vi "RP Lock-in Test.vi"() -> ()   [LabVIEW 2016]
uses:
  Instruments/Instrument Driver/Lock-in Driver/Lock-in Configuration.ctl
  Red Pitaya Lock-in Driver.lvclass
  C:/github/NHMFL_Core/Libraries/Instruments/Instrument Driver/Lock-in Driver/Lock-in Driver.lvclass
  C:/github/NHMFL_Core/Libraries/Instruments/Instrument Driver/Instrument Driver.lvclass
  Instruments/Instrument Driver/Instrument Driver.lvclass/Instrument Driver.ctl
  Red Pitaya Lock-in Driver.lvclass/Red Pitaya Lock-in Driver.ctl
  Instruments/Instrument Driver/Read Cycle period.vi
  Instruments/Instrument Driver/Read Group name.vi
  Instruments/Instrument Driver/Read Channel names.vi
  Instruments/Instrument Driver/Write Recorder name.vi
  Instruments/Instrument Driver/Write Cycle period.vi
  Read RP Instrument.vi
  Write RP Instrument.vi
  Instruments/Instrument Driver/Lock-in Driver/Write Lock-in configuration.vi
  RP Instrument/Write Server address.vi
  RP Instrument/Write Client type.vi
  Instruments/Instrument Driver/Lock-in Driver/Read Lock-in configuration.vi
  RP Instrument/RP Instrument.lvclass
  Instruments/Results/Acquired Result/Acquired Result.lvclass
panel:
  in  "Save result":bool
  in  "File Path Control":path=path "C:/Data/RPtest.tdms"
  out "XY Graph":cluster{dbl[], dbl[]}[](graph)
  in  "Update period":dbl=0.001 format="%#_6ps"
  in  "Lock-in configuration":T1={"Frequency"=0.0, "Time constant"=0.001, "Synchronous"=FALSE, "Channels"=[1]} {"Time constant" format="%#_6ps"; "Frequency" format="%#_6pHz"}
  in  "Start":dbl=1000.0 format="%#_6pHz"
  in  "End":dbl=10000000.0 format="%#_6pHz"
  in  "Step":dbl=10000.0 format="%#_6pHz"
  in  "Server address":string="192.168.1.100"
  out "Error Out":errorcluster
  in  "Error In":errorcluster
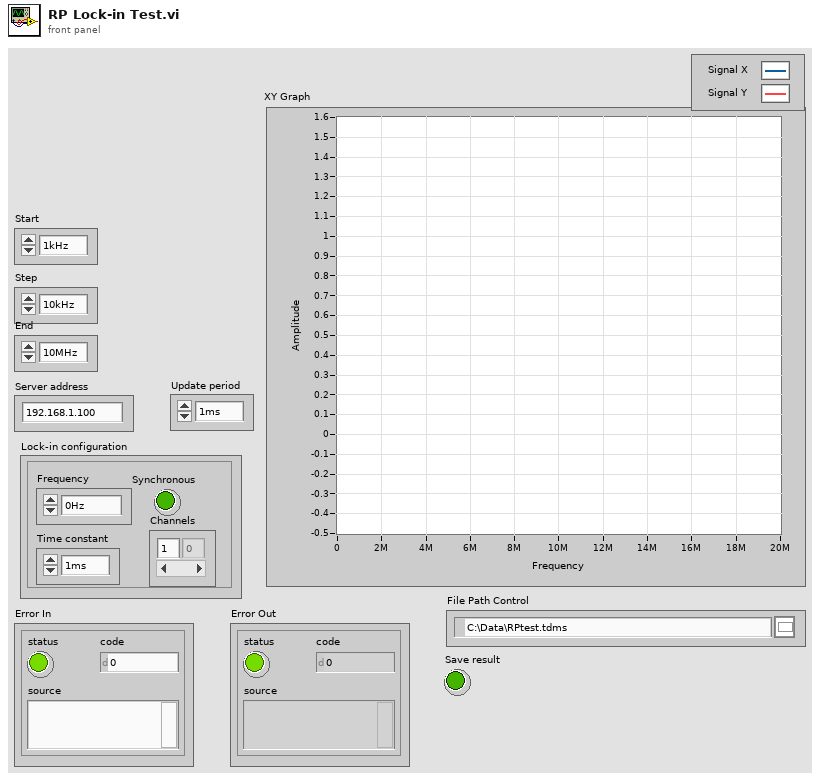
[diagram p1: front panel]
types:
  T1 = typedef "Lock-in Configuration.ctl" = cluster{"Frequency":dbl, "Time constant":dbl, "Synchronous":bool, "Channels":i32[]}
  T2 = enum16{"open", "open or create", "create or replace", "create", "open (read-only)"}
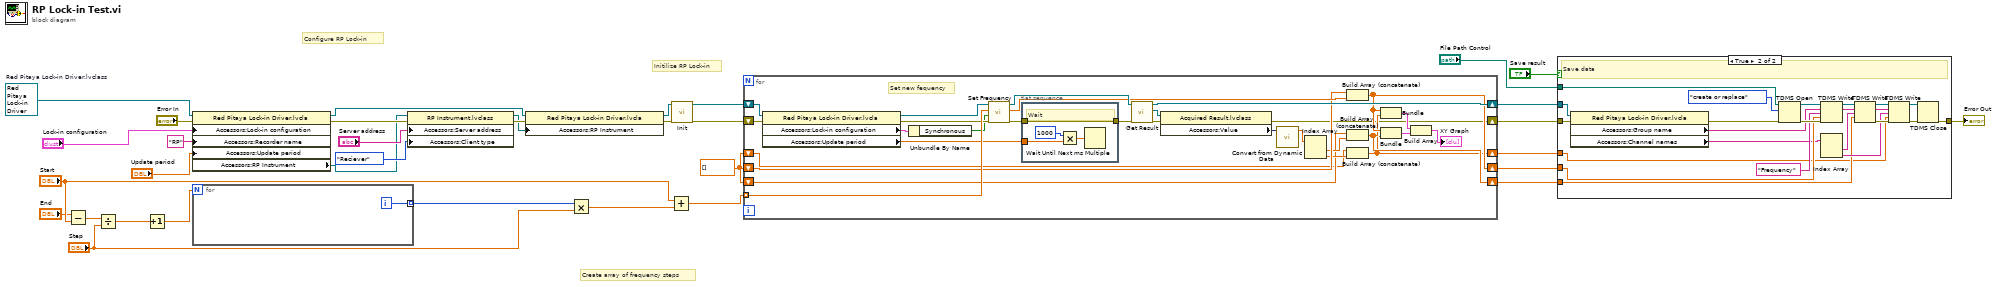
[diagram p0: block diagram]
diagram:
  w9 = dbl[] []
  w33 = refnum<class "Red Pitaya Lock-in Driver.lvclass"> refnum  # Red Pitaya Lock-in Driver.lvclass
  # "Initilize RP Lock-in"
  # "Configure RP Lock-in"
  # "Create array of frequency steps"
  n1 = Subtract(x="End", y="Start") -> (x-y=w20:dbl)
  n2 = Divide(x=w20, y="Step") -> (x/y=w21:dbl)
  n3 = Increment(x=w21) -> (x+1=w22:dbl)
  n4 = property class="Red Pitaya Lock-in Driver.lvcla"(reference=w33, error in="Error In", "Accessors:Lock-in configuration"="Lock-in configuration", "Accessors:Recorder name"="RP" ("Recorder name"), "Accessors:Update period"="Update period") -> (reference out=w29:refnum<class "Red Pitaya Lock-in Driver.lvclass">, error out=w31:errorcluster, "Accessors:RP Instrument"=w13:refnum<class "RP Instrument.lvclass">)
  n5 = for {
    N: w22 -> [_]
    tunnel: [w35] -> w23 mode=indexing
    i -> [w35]
  }
  n6 = property class="RP Instrument.lvclass"(reference=w13, error in=w31, "Accessors:Server address"="Server address", "Accessors:Client type"=enum16{"Control", "Reciever", "Transmitter"}."Reciever" ("Client type")) -> (reference out=w30:refnum<class "RP Instrument.lvclass">, error out=w32:errorcluster)
  n7 = property class="Red Pitaya Lock-in Driver.lvcla"(reference=w29, error in=w32, "Accessors:RP Instrument"=w30) -> (reference out=w16:refnum<class "Red Pitaya Lock-in Driver.lvclass">, error out=w17:errorcluster)
  n8 = Multiply(x=w23, y="Step") -> (x*y=w25:dbl[])
  n9 = Add(x="Start", y=w25) -> (x+y=w18:dbl[])
  n10 = call-dynamic "Init.vi"("error in (no error)"=w17, "Instrument Driver in"=w16) -> ("error out"=w14:errorcluster, "Instrument Driver out"=w15:refnum<class "Red Pitaya Lock-in Driver.lvclass">)  [unwired: 7 in, 1 out]
  n11 = for {
    tunnel: w18 -> [w64] mode=indexing
    shift-right: [w36] -> w7
    shift-left: w14 -> [w63]
    shift-right: [w52] -> w5
    shift-left: w15 -> [w61]
    shift-right: [w45] -> w4
    shift-left: w9 -> [w46]
    shift-right: [w38] -> w3
    shift-left: w9 -> [w40]
    shift-right: [w37] -> w2
    shift-left: w9 -> [w39]
    # "Set new fequency"
    n12 = property class="Red Pitaya Lock-in Driver.lvcla"(reference=w61, error in=w63) -> (reference out=w60:refnum<class "Red Pitaya Lock-in Driver.lvclass">, error out=w62:errorcluster, "Accessors:Lock-in configuration"=w59:T1, "Accessors:Update period"=w57:dbl)
    n13 = Unbundle By Name(w59) -> ("Synchronous"=w58:bool)
    n14 = call-dynamic "Set Frequency.vi"("error in (no error)"=w62, "Synchronous"=w58, "Frequency"=w64, "Red Pitaya Lock-in Driver in"=w60) -> ("error out"=w56:errorcluster, "Actual frequency"=w47:dbl, "Red Pitaya Lock-in Driver out"=w54:refnum<class "Red Pitaya Lock-in Driver.lvclass">)  [unwired: 5 in]
    n15 = flat-sequence {
      tunnel: w57 -> [w68]
      tunnel: w56 -> [w65]
      tunnel: [w65] -> w55
      frame #0 {
        # "Wait"
        n16 = Multiply(x=1000, y=w68) -> (x*y=w67:dbl)
        n17 = Wait Until Next ms Multiple(millisecond multiple=w67) -> ()  [unwired: 1 out]
      }
    }
    n18 = call-dynamic "Get Result.vi"("error in (no error)"=w55, "Red Pitaya Lock-in Driver in"=w54) -> ("error out"=w51:errorcluster, "Result"=w53:refnum<class "Acquired Result.lvclass">, "Red Pitaya Lock-in Driver out"=w52:refnum<class "Red Pitaya Lock-in Driver.lvclass">)  [unwired: 7 in]
    n19 = property class="Acquired Result.lvclass"(reference=w53, error in=w51) -> (error out=w36:errorcluster, "Accessors:Value"=w50:dynamicdata)  [unwired: 1 out]
    n20 = call "Convert from Dynamic Data"("Dynamic Data Type"=w50) -> ("Array"=w48:dbl[])  [unwired: 3 in]
    n21 = Index Array(array=w48) -> (element #1=w41:dbl, element #2=w42:dbl)  [unwired: 2 in]
    n22 = Build Array (concatenate)(w46, w47) -> (w45:dbl[])
    n23 = Build Array (concatenate)(w40, w41) -> (w38:dbl[])
    n24 = Build Array (concatenate)(w39, w42) -> (w37:dbl[])
    n25 = Bundle(w45, w38) -> (w44:cluster{dbl[], dbl[]})  [unwired: 1 in]
    n26 = Bundle(w45, w37) -> (w43:cluster{dbl[], dbl[]})  [unwired: 1 in]
    n27 = Build Array(w44, w43) -> (→"XY Graph":cluster{dbl[], dbl[]}[])
  }
  n28 = case shown="True" "Save result" {
    tunnel: "File Path Control" -> [_ w92]
    tunnel: w7 -> [w69 w74]
    tunnel: w5 -> [_ w88]
    tunnel: w4 -> [_ w80]
    tunnel: w3 -> [_ w76]
    tunnel: w2 -> [_ w75]
    tunnel: [w69 w70] -> w1
    frame False {
    }
    frame True {
      # "Save data"
      n29 = property class="Red Pitaya Lock-in Driver.lvcla"(reference=w88, error in=w74) -> (error out=w73:errorcluster, "Accessors:Group name"=w83:string, "Accessors:Channel names"=w79:string[])  [unwired: 1 out]
      n30 = TDMS Open(8:w73, 10:T2."create or replace" ("operation (0:open)"), 11:w92) -> (0:w90:errorcluster, 3:w89:refnum<k34>)  [unwired: 4 in]
      n31 = TDMS Write(0:w89, 5:w83, 7:"Frequency", 9:w80, 11:w90) -> (4:w84:refnum<k34>, 6:w82:string)  [unwired: 1 in, 2 out]
      n32 = Index Array(array=w79) -> (element #1=w78:string, element #2=w77:string)  [unwired: 2 in]
      n33 = TDMS Write(0:w84, 5:w82, 7:w78, 9:w76) -> (4:w87:refnum<k34>, 6:w86:string, 15:w85:errorcluster)  [unwired: 2 in, 1 out]
      n34 = TDMS Write(0:w87, 5:w86, 7:w77, 9:w75, 11:w85) -> (4:w71:refnum<k34>, 15:w72:errorcluster)  [unwired: 1 in, 2 out]
      n35 = TDMS Close(8:w72, 11:w71) -> (0:w70:errorcluster)  [unwired: 1 out]
    }
  }
  "Error Out" <- w1
